vi "TimerTest.vi"() -> ()   [LabVIEW 2016]
uses:
  APIs/Stimulus/VI/MakeVIFrontMost.vi
  APIs/Stimulus/ControlValue/ValueSignalLatchBooleanString.vi
  APIs/Assert/AssertControlValue/AlmostEqual.vi
  <vilib>/addons/_JKI Toolkits/Caraya/classes/Assert/Assert Almost Equal_Float.vi
  APIs/Stimulus/ControlValue/SetValueAuto.vi
  <vilib>/addons/_JKI Toolkits/Caraya/classes/Test/Test.lvclass
  Drona.lvlib
  APIs/Assert/AssertControlValue/AssertControlValue.lvlib
  APIs/Stimulus/ControlValue/ControlValue.lvlib
  <vilib>/addons/_JKI Toolkits/Caraya/classes/Assert/Assert.lvclass
  APIs/Stimulus/VI/VI.lvlib
panel:
  out "error out":errorcluster
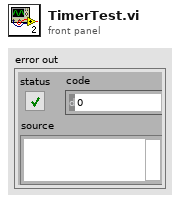
[diagram p1: front panel]
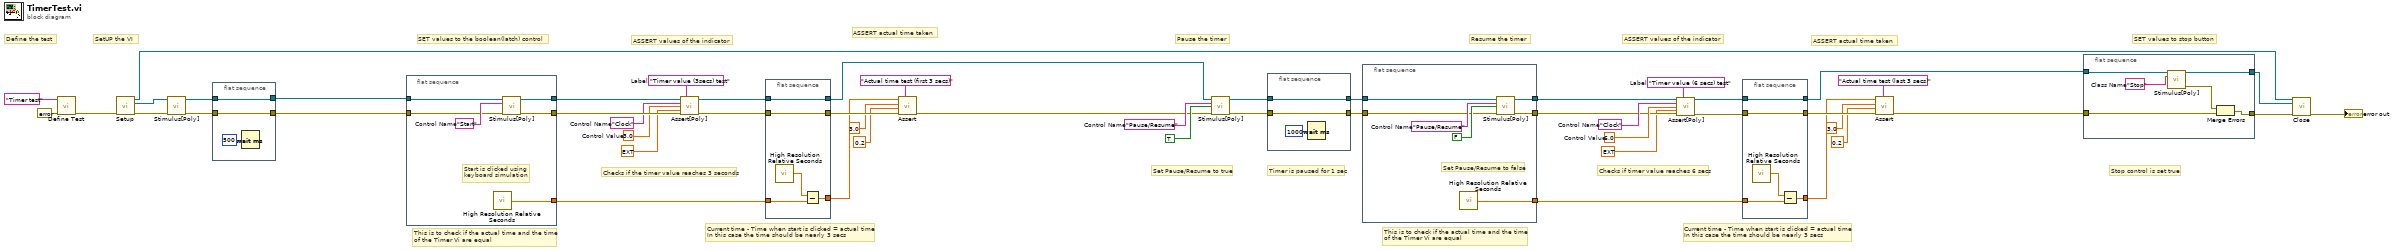
[diagram p0: block diagram]
diagram:
  w41 = "Clock"  # Control Name
  w42 = "Timer value (6 secs) test"  # Label
  w43 = 6.0  # Control Value
  w44 = "Pause/Resume"  # Control Name
  w45 = "Clock"  # Control Name
  w46 = "Timer value (3secs) test"  # Label
  w47 = 3.0  # Control Value
  # "ASSERT actual time taken"
  # "This is to check if the actual time and the time \nof the Timer Vi are equal"
  # "Current time - Time when start is clicked = actual time\nIn this case the time should be nearly 3 secs"
  # "ASSERT actual time taken"
  # "Current time - Time when start is clicked = actual time\nIn this case the time should be nearly 3 secs"
  # "This is to check if the actual time and the time \nof the Timer Vi are equal"
  # "Resume the timer"
  # "Timer is paused for 1 sec"
  # "Checks if timer value reaches 6 secs"
  # "ASSERT values of the indicator"
  # "Stop control is set true"
  # "SET values to stop button"
  # "Set Pause/Resume to true"
  # "Pause the timer"
  # "Checks if the timer value reaches 3 seconds"
  # "ASSERT values of the indicator"
  # "SET values to the boolean(latch) control"
  # "SetUP the VI"
  # "Define the test"
  n1 = call <vilib>:"Define Test.vi"("error in (no error)"=errorcluster {"status"=FALSE, "code"=0, "source"=""}, "Label (VI Title)"="Timer test") -> ("error out"=w7:errorcluster)  [unwired: 9 in]
  n2 = call "Setup.vi"("error in"=w7) -> ("Application Ref"=w3:refnum<vi>, "VI Reference Out"=w2:refnum<vi>, "error out"=w1:errorcluster)  [unwired: 12 in]
  n3 = call-poly "Stimulus[Poly].vi"("VI Reference In"=w2, "error in"=w1) -> ("VI Reference Out"=w8:refnum<vi>, "error out"=w11:errorcluster)  [unwired: 12 in]
  n4 = flat-sequence {
    tunnel: w11 -> [w53]
    tunnel: [w53] -> w10
    tunnel: [w52] -> w9
    tunnel: w8 -> [w52]
    frame #0 {
      n5 = Wait (ms)(milliseconds to wait=u32 500) -> ()  [unwired: 1 out]
    }
  }
  n6 = flat-sequence {
    tunnel: [w60] -> w49
    tunnel: [w59] -> w48
    tunnel: w10 -> [w57]
    tunnel: w9 -> [w55]
    tunnel: [w56] -> w27
    frame #0 {
      w58 = "Start"  # Control Name
      # "Start is clicked using \nkeyboard simulation"
      n7 = call <vilib>:"High Resolution Relative Seconds.vi"() -> ("relative seconds"=w56:dbl)
      n8 = call-poly "Stimulus[Poly].vi"("VI Reference In"=w55, "Control Path"=w58, "error in"=w57) -> ("VI Reference Out"=w59:refnum<vi>, "error out"=w60:errorcluster)  [unwired: 11 in]
    }
  }
  n9 = call-poly "Assert[Poly].vi"("VI Reference In"=w48, "Label"=w46, "Control Path"=w45, "Control Value"=w47, "Tolerance"=ext 0.2, "Error In"=w49) -> ("VI Reference Out"=w29:refnum<vi>, "Error Out"=w31:errorcluster)  [unwired: 8 in]
  n10 = flat-sequence {
    tunnel: w31 -> [w65]
    tunnel: [w65] -> w30
    tunnel: w29 -> [w64]
    tunnel: [w64] -> w28
    tunnel: w27 -> [w62]
    tunnel: [w63] -> w25
    frame #0 {
      n11 = call <vilib>:"High Resolution Relative Seconds.vi"() -> ("relative seconds"=w61:dbl)
      n12 = Subtract(x=w61, y=w62) -> (x-y=w63:dbl)
    }
  }
  n13 = call-poly <vilib>:"Assert.vi"("Label"="Actual time test (first 3 secs)", "error in (no error)"=w30, "Tolerance"=0.2, "Y"=3.0, "X"=w25) -> ("error out"=w26:errorcluster)  [unwired: 6 in]
  n14 = call-poly "Stimulus[Poly].vi"("VI Reference In"=w28, "Control Path"=w44, "Value (Signaling)"=TRUE, "error in"=w26) -> ("VI Reference Out"=w37:refnum<vi>, "error out"=w38:errorcluster)  [unwired: 10 in]
  n15 = flat-sequence {
    tunnel: w38 -> [w67]
    tunnel: [w67] -> w35
    tunnel: w37 -> [w66]
    tunnel: [w66] -> w36
    frame #0 {
      n16 = Wait (ms)(milliseconds to wait=u32 1000) -> ()  [unwired: 1 out]
    }
  }
  n17 = flat-sequence {
    tunnel: w36 -> [w73]
    tunnel: w35 -> [w72]
    tunnel: [w71] -> w34
    tunnel: [w70] -> w33
    tunnel: [w69] -> w15
    frame #0 {
      w74 = "Pause/Resume"  # Control Name
      # "Set Pause/Resume to false"
      n18 = call <vilib>:"High Resolution Relative Seconds.vi"() -> ("relative seconds"=w69:dbl)
      n19 = call-poly "Stimulus[Poly].vi"("VI Reference In"=w73, "Control Path"=w74, "Value (Signaling)"=FALSE, "error in"=w72) -> ("VI Reference Out"=w70:refnum<vi>, "error out"=w71:errorcluster)  [unwired: 10 in]
    }
  }
  n20 = call-poly "Assert[Poly].vi"("VI Reference In"=w33, "Label"=w42, "Control Path"=w41, "Control Value"=w43, "Tolerance"=ext 0.2, "Error In"=w34) -> ("VI Reference Out"=w14:refnum<vi>, "Error Out"=w16:errorcluster)  [unwired: 8 in]
  n21 = flat-sequence {
    tunnel: w16 -> [w80]
    tunnel: [w80] -> w21
    tunnel: w14 -> [w79]
    tunnel: [w79] -> w13
    tunnel: w15 -> [w77]
    tunnel: [w78] -> w20
    frame #0 {
      n22 = call <vilib>:"High Resolution Relative Seconds.vi"() -> ("relative seconds"=w76:dbl)
      n23 = Subtract(x=w76, y=w77) -> (x-y=w78:dbl)
    }
  }
  n24 = call-poly <vilib>:"Assert.vi"("Label"="Actual time test (last 3 secs)", "error in (no error)"=w21, "Tolerance"=0.2, "Y"=3.0, "X"=w20) -> ("error out"=w12:errorcluster)  [unwired: 6 in]
  n25 = flat-sequence {
    tunnel: [w84] -> w5
    tunnel: [w85] -> w6
    tunnel: w13 -> [w83]
    tunnel: w12 -> [w81]
    frame #0 {
      w86 = "Stop"  # Class Name
      n26 = call-poly "Stimulus[Poly].vi"("VI Reference In"=w83, "Control Path"=w86) -> ("VI Reference Out"=w85:refnum<vi>, "error out"=w82:errorcluster)  [unwired: 12 in]
      n27 = Merge Errors(w82, w81) -> (w84:errorcluster)
    }
  }
  n28 = call "Close.vi"("Application Ref"=w3, "VI Reference Out"=w6, "error in"=w5) -> ("error out"=→"error out":errorcluster)  [unwired: 12 in]
